vi "Conductus Ramp Temperature.vi"(2 "Point #":i32, 4 "Parameters":dbl[](array[numeric]) format="%.3e", 5 "Instrument Address":refnum<visa-resource-name>) -> (0 "Stop":bool, 1 "Data Out":dbl[](array[numeric]) format="%.2e")   [LabVIEW 2020]
doc: "This VI ramps the setpoint of the Conductus LTC 20 temperature controller at a set rate. The set point rate is calculated asynchronously from the time since the index was <= 0.\nScott Hannahs, NHMFL - FSU, Feb 1996"
panel:
  # "Starting Temp"
  # "Ending Temp"
  # "Time (Min)"
  # "Set Point"
  # "Heater Power"
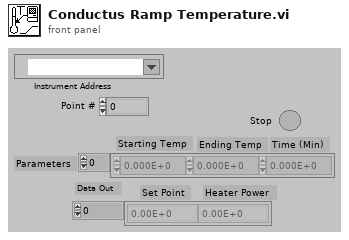
[diagram p1: front panel]
types:
  T1 = cluster{"Parameters[0]":dbl, "Parameters[1]":dbl, "Parameters[2]":dbl}
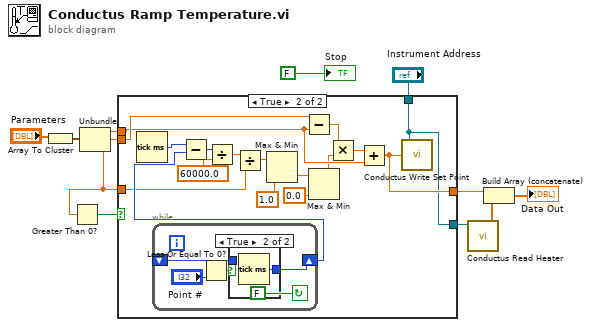
[diagram p0: block diagram]
diagram:
  n1 = Array To Cluster(array="Parameters") -> (cluster=w8:T1)
  n2 = Unbundle(w8) -> ("Parameters[0]"=w6:dbl, "Parameters[1]"=w7:dbl, "Parameters[2]"=w10:dbl)
  n3 = Greater Than 0?(x=w10) -> (x > 0?=w12:bool)
  n4 = case shown="True" w12 {
    tunnel: w10 -> [_ w26]
    tunnel: "Instrument Address" -> [w13 w15]
    tunnel: w7 -> [_ w21]
    tunnel: w6 -> [w14 w20]
    tunnel: [w14 w16] -> w4
    tunnel: [w13 w15] -> w2
    frame False {
    }
    frame True {
      n5 = Tick Count (ms)() -> (millisecond timer value=w31:u32)
      n6 = while {
        shift-left: _ -> [w33]
        shift-right: [w34] -> w30
        stop <- FALSE continue-if-true
        n7 = Less Or Equal To 0?(x="Point #") -> (x <= 0?=w35:bool)
        n8 = case shown="True" w35 {
          tunnel: [w37 w38] -> w34
          tunnel: w33 -> [w37 _]
          frame False {
          }
          frame True {
            n9 = Tick Count (ms)() -> (millisecond timer value=w38:u32)
          }
        }
      }
      n10 = Subtract(x=w31, y=w30) -> (x-y=w29:u32)
      n11 = Divide(x=w29, y=60000.0) -> (x/y=w27:dbl)
      n12 = Divide(x=w27, y=w26) -> (x/y=w24:dbl)
      n13 = Max & Min(x=w24, y=1.0) -> (min(x,y)=w18:dbl)  [unwired: 1 out]
      n14 = Subtract(x=w21, y=w20) -> (x-y=w25:dbl)
      n15 = Max & Min(x=w18, y=0.0) -> (max(x,y)=w19:dbl)  [unwired: 1 out]
      n16 = Multiply(x=w25, y=w19) -> (x*y=w23:dbl)
      n17 = Add(x=w23, y=w20) -> (x+y=w16:dbl)
      n18 = call "Conductus Write Set Point.vi"("Setpoint"=w16, "Instrument Address"=w15) -> ()  [unwired: 1 in]
    }
  }
  n19 = call "Conductus Read Heater.vi"("Instrument Address"=w2) -> ("Heater Power %"=w5:dbl[])
  n20 = Build Array (concatenate)(w4, w5) -> (→"Data Out":dbl[])
  "Stop" <- FALSE
